vi "Read Multiple Analog Channels.vi"() -> ()   [LabVIEW 2020]
uses:
  <instrlib>/BDAQ-6104/BDAQ-6104.lvlib
panel:
  out "Channel Data":dbl[](array[numeric])
  in  "VISA resource name":refnum<visa-resource-name>
  in  "Channel Selection":T1(array[ring])=[enum."Channel 0", enum."Channel 1"]
  # "Volts"
  # "Read the specified analog channel values. The default\ndata value is in volts."
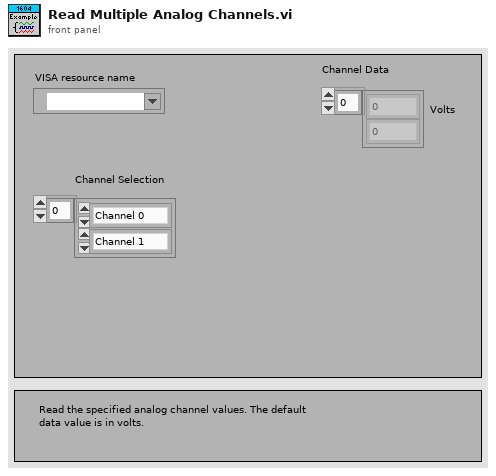
[diagram p1: front panel]
types:
  T1 = enum16{"Channel 0", "Channel 1", "Channel 2", "Channel 3", "Channel 4", "Channel 5"}[]
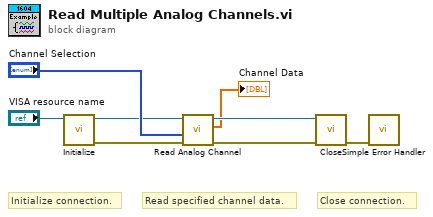
[diagram p0: block diagram]
diagram:
  # "Close connection."
  # "Read specified channel data."
  # "Initialize connection."
  n1 = call <instrlib>:"Initialize.vi"("VISA resource name"="VISA resource name") -> ("error out"=w8:errorcluster, "VISA resource name out"=w6:refnum<visa-resource-name>)  [unwired: 9 in]
  n2 = call-poly <instrlib>:"Read Analog Channel.vi"("error in"=w8, "Channel Selection"="Channel Selection", "VISA resource name"=w6) -> ("error out"=w4:errorcluster, "Channel Data"=→"Channel Data":dbl[], "VISA resource name"=w3:refnum<visa-resource-name>)  [unwired: 6 in]
  n3 = call <instrlib>:"Close.vi"("error in (no error)"=w4, "VISA resource name"=w3) -> ("error out"=w1:errorcluster)  [unwired: 9 in]
  n4 = call <vilib>:"Simple Error Handler.vi"("error in (no error)"=w1) -> ()  [unwired: 4 in, 5 out]
